vi "setTimerResolution.vi"(8 "error in (no error)":errorcluster, 10 "resolution":T1, 11 "CCD in":refnum<class "CCD.lvclass">) -> (0 "error out":errorcluster, 1 "ID":i32, 2 "results-JSON string":string, 3 "CCD out":refnum<class "CCD.lvclass">)   [LabVIEW 2023, in "CCD.lvclass"]
uses:
  CCD.lvclass
  CCD.lvclass/CCD.ctl
  20f7d3bd-08ac-4524-9bed-df36c1da25a0.vi
  GenericDevice/GenericDevice.lvclass
  <vilib>/IlluminatedG/lv-web-crypto/lv-json/JSON/JSON.lvlib
  2615cbe5-8692-4f73-8789-456f633c95b5.vi
  TimerResolutionEnum.ctl
panel:
  # "Connector Pane"
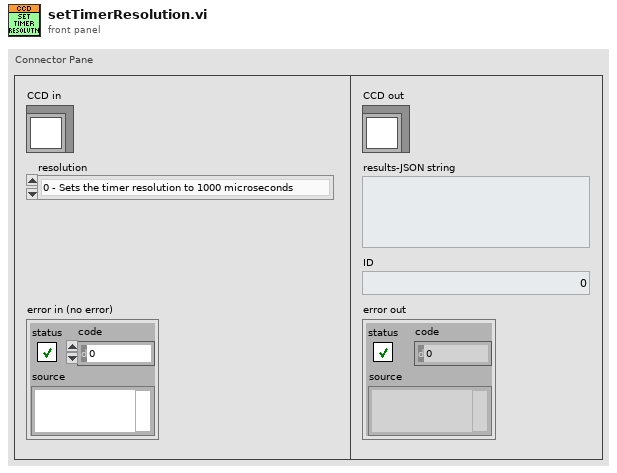
[diagram p1: front panel]
types:
  T1 = typedef "CCD.lvclass/TimerResolutionEnum.ctl" = enum16{"0 - Sets the timer resolution to 1000 microseconds", "1 - Sets the timer resolution to 1 microsecond"}
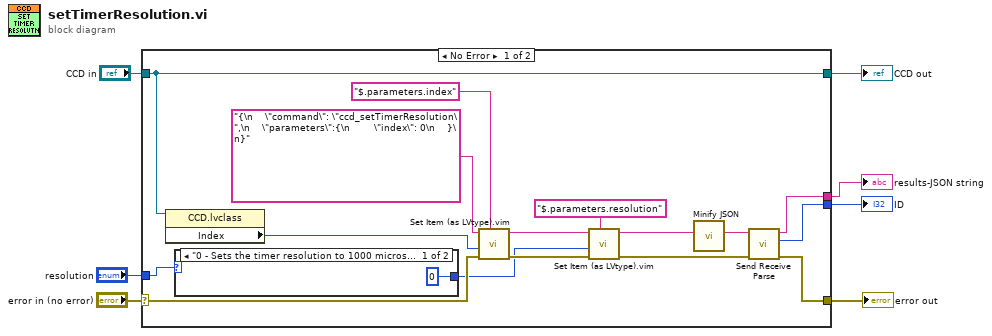
[diagram p0: block diagram]
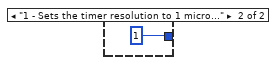
[diagram p2: hidden frame]
diagram:
  n1 = case shown="No Error" "error in (no error)" {
    selector: "error in (no error)" -> [w19 w27]
    tunnel: [w18 w27] -> w6
    tunnel: [w21 w26] -> w4
    tunnel: "CCD in" -> [w21 w26]
    tunnel: [w17 _] -> w3
    tunnel: [w16 _] -> w2
    tunnel: "resolution" -> [w9 _]
    frame No Error {
      n2 = property class="CCD.lvclass"(reference=w21) -> ("Index"=w20:i32)  [unwired: 1 in, 2 out]
      n3 = case shown="\"0 - Sets the timer resolution to 1000 microseconds\", Default" w9 {
        tunnel: [0 1] -> w8
        frame "0 - Sets the timer resolution to 1000 microseconds", Default {
        }
        frame "1 - Sets the timer resolution to 1 microsecond" {
        }
      }
      n4 = call "Set Item (as LVtype).vim"("$Path or Item Name"="$.parameters.index", "error in (no error)"=w19, "Anything"=w20, "JSON"="{\n    \"command\": \"ccd_setTimerResolution\",\n    \"parameters\":{\n        \"index\": 0\n    }\n}") -> ("error out"=w11:errorcluster, "<JSON>"=w13:string)  [unwired: 4 in, 1 out]
      n5 = call "Set Item (as LVtype).vim"("$Path or Item Name"="$.parameters.resolution", "error in (no error)"=w11, "Anything"=w8, "JSON"=w13) -> ("error out"=w10:errorcluster, "<JSON>"=w12:string)  [unwired: 4 in, 1 out]
      n6 = call <vilib>:"Minify JSON.vi"("JSON String"=w12) -> ("Minified JSON"=w15:string)  [unwired: 10 in]
      n7 = call "Send Receive Parse.vi"("error in"=w10, "<JSON>"=w15) -> ("error out"=w18:errorcluster, "ID"=w16:i32, "results-JSON string"=w17:string)  [unwired: 7 in]
    }
    frame Error {
    }
  }
  "error out" <- w6
  "CCD out" <- w4
  "results-JSON string" <- w3
  "ID" <- w2
